vi "Lab Panel V5.40.vi"() -> ()   [LabVIEW 2017] (continued)
                          }
                        }
                      }
                    }
                  }
                }
              }
              event "RUN LAB01-2": Value Change {
                n584 = event-data() -> ("NewVal"=w850:bool)  [unwired: 1 in, 5 out]
                n585 = local write "run lab01-2"(w850) -> ()
                n586 = case shown="True" w850 {
                  tunnel: w856 -> [_ w894]
                  tunnel: w855 -> [_ w893]
                  tunnel: w853 -> [w858 w892]
                  tunnel: w854 -> [_ w891]
                  tunnel: w852 -> [_ w890]
                  tunnel: [w857 w889] -> w851
                  tunnel: w849 -> [_ w888]
                  tunnel: w848 -> [_ w887]
                  tunnel: w847 -> [_ w886]
                  tunnel: w846 -> [_ w884]
                  frame False {
                    # "stop test"
                    n587 = stacked-sequence {
                      tunnel: w858 -> [w867 _]
                      tunnel: [w859 _] -> w857
                      frame #0 {
                        n588 = local read "DISP LAB01-2"() -> (w866:T4)
                        n589 = Unbundle(w866) -> ("CYCLE"=w864:dbl, "MINS"=w865:dbl)  [unwired: 1 out]
                        n590 = case shown="\"CHART TEST\", Default" w867 {
                          tunnel: w865 -> [_ _ w874]
                          tunnel: w864 -> [w872 w873 _]
                          tunnel: [w872 w873 w874] -> w863
                          frame "CHART TEST", Default {
                          }
                          frame "CYCLE TEST" {
                          }
                          frame "T-RISE TEST" {
                          }
                        }
                        n591 = local read "TDMS LAB01-2"() -> (w871:refnum<k34>)
                        n592 = Build Array("STOPPED") -> (w868:string[])
                        n593 = Build Array(w863) -> (w862:dbl[])
                        n594 = TDMS Write(0:w871, 5:"TEST RESULT", 7:w868, 9:w862) -> (4:w860:refnum<k34>, 15:w861:errorcluster)  [unwired: 2 in, 2 out]
                        n595 = TDMS Close(8:w861, 11:w860) -> (0:w859:errorcluster)  [unwired: 1 out]
                      }
                      frame #1 {
                        n596 = local read "DISP LAB01-2"() -> (w878:T4)
                        n597 = stacked-sequence {
                          tunnel: "LAB01-2" -> [w880 w882]
                          frame #0 {
                            n598 = call "sub vi - defrag tdms v1.vi"("panel id"=w880) -> ("error out"=w879:errorcluster)  [unwired: 10 in]
                            n599 = local write "data file error"(w879) -> ()
                          }
                          frame #1 {
                            n600 = call "Save data file (stop) v3.vi"("panel id"=w882) -> ("network file save error"=w881:errorcluster)  [unwired: 9 in, 1 out]
                            n601 = local write "RESULT LAB01-2"(FALSE) -> ()
                            n602 = local write "data file error"(w881) -> ()
                          }
                        }
                        n603 = Bundle(cluster=w878, "STATUS"="STOP") -> (w876:T4)  [unwired: 2 in]
                        n604 = local write "DISP LAB01-2"(w876) -> ()
                      }
                    }
                  }
                  frame True {
                    n605 = local read "SIG LAB01-2"() -> (w885:T2)
                    n606 = stacked-sequence {
                      seq-local: [w896 _] -> [_ w900]
                      tunnel: w894 -> [_ w910]
                      tunnel: w893 -> [_ w909]
                      tunnel: w892 -> [_ w908]
                      tunnel: w891 -> [_ w907]
                      tunnel: w890 -> [_ w906]
                      tunnel: [_ w905] -> w889
                      tunnel: w888 -> [_ w904]
                      tunnel: w887 -> [_ w903]
                      tunnel: w886 -> [_ w902]
                      tunnel: w885 -> [w895 w901]
                      tunnel: w884 -> [_ w899]
                      frame #0 {
                        n607 = Unbundle(w895) -> ("AMPS"=w898:dbl)  [unwired: 4 out]
                        n608 = call "Check For Amps on v1.vi"("ID"="LAB01-2", "amps"=w898) -> ("amps"=w896:bool)  [unwired: 9 in]
                      }
                      frame #1 {
                        n609 = case shown="True" w900 {
                          tunnel: w910 -> [_ w923]
                          tunnel: w909 -> [_ w922]
                          tunnel: w908 -> [_ w921]
                          tunnel: w907 -> [_ w920]
                          tunnel: w906 -> [_ w919]
                          tunnel: [errorcluster {"status"=FALSE, "code"=0, "source"=""} ("error out") w918] -> w905
                          tunnel: w904 -> [_ w917]
                          tunnel: w903 -> [_ w916]
                          tunnel: w902 -> [_ w915]
                          tunnel: w901 -> [_ w914]
                          tunnel: w899 -> [_ w913]
                          frame False {
                            w911 = FALSE
                            n610 = local write "RUN LAB01-2"(w911) -> ()
                            n611 = local write "run lab01-2"(w911) -> ()
                          }
                          frame True {
                            n612 = stacked-sequence {
                              seq-local: [w924 _ _ _ _] -> [_ w948 _ _ _]
                              tunnel: w923 -> [w929 _ _ _ _]
                              tunnel: w922 -> [w926 _ _ _ _]
                              tunnel: w921 -> [w939 _ _ _ _]
                              tunnel: w920 -> [w932 _ _ _ _]
                              tunnel: w919 -> [w927 _ _ _ _]
                              tunnel: [_ w943 _ _ _] -> w918
                              tunnel: w917 -> [_ _ _ w970 _]
                              tunnel: w916 -> [_ _ _ w969 _]
                              tunnel: w915 -> [_ _ _ w968 _]
                              tunnel: w914 -> [_ _ _ _ _]
                              tunnel: w913 -> [_ _ _ _ w983]
                              frame #0 {
                                w925 = "\\"
                                n613 = local read "SET LAB01-2"() -> (w934:T5)
                                n614 = case shown="\"CYCLE TEST\"" w939 {
                                tunnel: ["L01-2-CHART TEST-" "L01-2-CYCLE TEST-" "L01-2-T-RISE TEST-"] -> w935
                                frame "CHART TEST", Default {
                                }
                                frame "CYCLE TEST" {
                                }
                                frame "T-RISE TEST" {
                                }
                                }
                                n615 = Unbundle(w934) -> ("DESCRIPTION"=w933:string)  [unwired: 4 out]
                                n616 = Concatenate Strings(w929, "\\", w927, w925, w926, w925) -> (w936:string)
                                n617 = String To Path(string=w936) -> (path=w938:path)
                                n618 = Concatenate Strings(w936, w935, w933, "-", w932, ".tdms") -> (w924:string)
                                n619 = Create Folder(path (use dialog)=w938) -> (error out=w937:errorcluster)  [unwired: 2 in, 2 out]
                                n620 = call <vilib>:"Clear Errors.vi"("error in (no error)"=w937) -> ()  [unwired: 5 in, 2 out]
                                n621 = global write "Global 1.vi" "LAB01-2 FILE"(w924) -> ()
                              }
                              frame #1 {
                                (unwired) FALSE
                                n622 = String To Path(string=w948) -> (path=w944:path)
                                n623 = TDMS Open(6:FALSE, 10:T22."create or replace" ("operation (0:open)"), 11:w944) -> (0:w943:errorcluster, 3:→"TDMS LAB01-2":refnum<k34>)  [unwired: 4 in]
                              }
                              frame #2 {
                                n624 = local read "SET LAB01-2"() -> (w954:T5)
                                n625 = local read "TDMS LAB01-2"() -> (w965:refnum<k34>)
                                n626 = Build Array("Testers Name", "Description", "Set Test Cycles", "T-Rise minutes", "T-Rise Deg C") -> (w955:string[])
                                n627 = Unbundle(w954) -> ("NAME"=w953:string, "DESCRIPTION"=w952:string, "CYCLES"=w951:dbl, "T-RISE mins"=w950:dbl, "T-RISE deg C"=w949:dbl)
                                n628 = Number To Decimal String(number=w951) -> (decimal integer string=w964:string)  [unwired: 1 in]
                                n629 = Number To Decimal String(number=w950) -> (decimal integer string=w963:string)  [unwired: 1 in]
                                n630 = Number To Decimal String(number=w949) -> (decimal integer string=w962:string)  [unwired: 1 in]
                                n631 = Build Array(w953, w952, w964, w963, w962) -> (w961:string[])
                                n632 = TDMS Set Properties(5:w961, 7:w955, 11:w965) -> ()  [unwired: 3 in, 4 out]
                              }
                              frame #3 {
                                n633 = local read "DISP LAB01-2"() -> (w967:T4)
                                n634 = Concatenate Strings("LAB01-2  ", w970) -> (w971:string)
                                n635 = Two Button Dialog(message=w971, 1:w968, 2:w969) -> (T button?=w973:bool)
                                n636 = case shown="True" w973 {
                                tunnel: w967 -> [w980 w981]
                                tunnel: [w980 w981] -> w977
                                tunnel: [w979 w982] -> w976
                                tunnel: [w978 w982] -> w975
                                frame False {
                                n637 = Unbundle(w980) -> ("CYCLE"=w979:dbl, "MINS"=w978:dbl)  [unwired: 1 out]
                                }
                                frame True {
                                w982 = 0.0
                                }
                                }
                                n638 = Bundle(cluster=w977, "CYCLE"=w976, "MINS"=w975, "STATUS"="RUN") -> (w966:T4)
                                n639 = local write "DISP LAB01-2"(w966) -> ()
                              }
                              frame #4 {
                                n640 = local read "TEMP START LAB01-2"() -> (w985:cluster{"TL":dbl, "TN":dbl})
                                n641 = Bundle(cluster=w985, "TL"=w983, "TN"=w983) -> (w984:cluster{"TL":dbl, "TN":dbl})
                                n642 = local write "TEMP START LAB01-2"(w984) -> ()
                              }
                            }
                          }
                        }
                      }
                    }
                  }
                }
              }
              event "RUN LAB02-1": Value Change {
                n643 = event-data() -> ("NewVal"=w991:bool)  [unwired: 1 in, 5 out]
                n644 = local read "SIG LAB02-1"() -> (w987:T2)
                n645 = case shown="True" w991 {
                  tunnel: w997 -> [_ w1035]
                  tunnel: w996 -> [_ w1034]
                  tunnel: w994 -> [w999 w1033]
                  tunnel: w995 -> [_ w1032]
                  tunnel: w993 -> [_ w1031]
                  tunnel: [w998 w1030] -> w992
                  tunnel: w990 -> [_ w1029]
                  tunnel: w989 -> [_ w1028]
                  tunnel: w988 -> [_ w1027]
                  tunnel: w987 -> [_ w1026]
                  tunnel: w986 -> [_ w1025]
                  frame False {
                    # "stop test"
                    n646 = stacked-sequence {
                      tunnel: w999 -> [w1008 _]
                      tunnel: [w1000 _] -> w998
                      frame #0 {
                        n647 = local read "DISP LAB02-1"() -> (w1007:T4)
                        n648 = Unbundle(w1007) -> ("CYCLE"=w1005:dbl, "MINS"=w1006:dbl)  [unwired: 1 out]
                        n649 = case shown="\"CYCLE TEST\"" w1008 {
                          tunnel: w1006 -> [_ _ w1015]
                          tunnel: w1005 -> [w1013 w1014 _]
                          tunnel: [w1013 w1014 w1015] -> w1004
                          frame "CHART TEST", Default {
                          }
                          frame "CYCLE TEST" {
                          }
                          frame "T-RISE TEST" {
                          }
                        }
                        n650 = local read "TDMS LAB02-1"() -> (w1012:refnum<k34>)
                        n651 = Build Array("STOPPED") -> (w1009:string[])
                        n652 = Build Array(w1004) -> (w1003:dbl[])
                        n653 = TDMS Write(0:w1012, 5:"TEST RESULT", 7:w1009, 9:w1003) -> (4:w1001:refnum<k34>, 15:w1002:errorcluster)  [unwired: 2 in, 2 out]
                        n654 = TDMS Close(8:w1002, 11:w1001) -> (0:w1000:errorcluster)  [unwired: 1 out]
                      }
                      frame #1 {
                        n655 = local read "DISP LAB02-1"() -> (w1019:T4)
                        n656 = stacked-sequence {
                          tunnel: "LAB02-1" -> [w1021 w1023]
                          frame #0 {
                            n657 = call "sub vi - defrag tdms v1.vi"("panel id"=w1021) -> ("error out"=w1020:errorcluster)  [unwired: 10 in]
                            n658 = local write "data file error"(w1020) -> ()
                          }
                          frame #1 {
                            n659 = local write "RESULT LAB02-1"(FALSE) -> ()
                            n660 = call "Save data file (stop) v3.vi"("panel id"=w1023) -> ("network file save error"=w1022:errorcluster)  [unwired: 9 in, 1 out]
                            n661 = local write "data file error"(w1022) -> ()
                          }
                        }
                        n662 = Bundle(cluster=w1019, "STATUS"="STOP") -> (w1017:T4)  [unwired: 2 in]
                        n663 = local write "DISP LAB02-1"(w1017) -> ()
                      }
                    }
                  }
                  frame True {
                    n664 = stacked-sequence {
                      seq-local: [w1037 _] -> [_ w1041]
                      tunnel: w1035 -> [_ w1051]
                      tunnel: w1034 -> [_ w1050]
                      tunnel: w1033 -> [_ w1049]
                      tunnel: w1032 -> [_ w1048]
                      tunnel: w1031 -> [_ w1047]
                      tunnel: [_ w1046] -> w1030
                      tunnel: w1029 -> [_ w1045]
                      tunnel: w1028 -> [_ w1044]
                      tunnel: w1027 -> [_ w1043]
                      tunnel: w1026 -> [w1036 w1042]
                      tunnel: w1025 -> [_ w1040]
                      frame #0 {
                        n665 = Unbundle(w1036) -> ("AMPS"=w1039:dbl)  [unwired: 4 out]
                        n666 = call "Check For Amps on v1.vi"("ID"="LAB02-1", "amps"=w1039) -> ("amps"=w1037:bool)  [unwired: 9 in]
                      }
                      frame #1 {
                        n667 = case shown="True" w1041 {
                          tunnel: w1051 -> [_ w1064]
                          tunnel: w1050 -> [_ w1063]
                          tunnel: w1049 -> [_ w1062]
                          tunnel: w1048 -> [_ w1061]
                          tunnel: w1047 -> [_ w1060]
                          tunnel: [errorcluster {"status"=FALSE, "code"=0, "source"=""} ("error out") w1059] -> w1046
                          tunnel: w1045 -> [_ w1058]
                          tunnel: w1044 -> [_ w1057]
                          tunnel: w1043 -> [_ w1056]
                          tunnel: w1042 -> [_ w1055]
                          tunnel: w1040 -> [_ w1054]
                          frame False {
                            w1053 = FALSE
                            n668 = local write "RUN LAB02-1"(w1053) -> ()
                            n669 = local write "run lab02-1"(w1053) -> ()
                          }
                          frame True {
                            n670 = stacked-sequence {
                              seq-local: [w1065 _ _ _ _] -> [_ w1089 _ _ _]
                              tunnel: w1064 -> [w1070 _ _ _ _]
                              tunnel: w1063 -> [w1067 _ _ _ _]
                              tunnel: w1062 -> [w1080 _ _ _ _]
                              tunnel: w1061 -> [w1073 _ _ _ _]
                              tunnel: w1060 -> [w1068 _ _ _ _]
                              tunnel: [_ w1084 _ _ _] -> w1059
                              tunnel: w1058 -> [_ _ _ w1110 _]
                              tunnel: w1057 -> [_ _ _ w1109 _]
                              tunnel: w1056 -> [_ _ _ w1108 _]
                              tunnel: w1055 -> [_ _ _ _ _]
                              tunnel: w1054 -> [_ _ _ _ w1124]
                              frame #0 {
                                w1066 = "\\"
                                n671 = local read "SET LAB02-1"() -> (w1075:T5)
                                n672 = case shown="\"CYCLE TEST\"" w1080 {
                                tunnel: ["L02-1-CHART TEST-" "L02-1-CYCLE TEST-" "L02-1-T-RISE TEST-"] -> w1076
                                frame "CHART TEST", Default {
                                }
                                frame "CYCLE TEST" {
                                }
                                frame "T-RISE TEST" {
                                }
                                }
                                n673 = Unbundle(w1075) -> ("DESCRIPTION"=w1074:string)  [unwired: 4 out]
                                n674 = Concatenate Strings(w1070, "\\", w1068, w1066, w1067, w1066) -> (w1077:string)
                                n675 = String To Path(string=w1077) -> (path=w1079:path)
                                n676 = Concatenate Strings(w1077, w1076, w1074, "-", w1073, ".tdms") -> (w1065:string)
                                n677 = Create Folder(path (use dialog)=w1079) -> (error out=w1078:errorcluster)  [unwired: 2 in, 2 out]
                                n678 = global write "Global 1.vi" "LAB02-1 FILE"(w1065) -> ()
                                n679 = call <vilib>:"Clear Errors.vi"("error in (no error)"=w1078) -> ()  [unwired: 5 in, 2 out]
                              }
                              frame #1 {
                                (unwired) FALSE
                                n680 = String To Path(string=w1089) -> (path=w1085:path)
                                n681 = TDMS Open(6:FALSE, 10:T22."create or replace" ("operation (0:open)"), 11:w1085) -> (0:w1084:errorcluster, 3:→"TDMS LAB02-1":refnum<k34>)  [unwired: 4 in]
                              }
                              frame #2 {
                                n682 = local read "SET LAB02-1"() -> (w1095:T5)
                                n683 = local read "TDMS LAB02-1"() -> (w1106:refnum<k34>)
                                n684 = Build Array("Testers Name", "Description", "Set Test Cycles", "T-Rise minutes", "T-Rise Deg C") -> (w1096:string[])
                                n685 = Unbundle(w1095) -> ("NAME"=w1094:string, "DESCRIPTION"=w1093:string, "CYCLES"=w1092:dbl, "T-RISE mins"=w1091:dbl, "T-RISE deg C"=w1090:dbl)
                                n686 = Number To Decimal String(number=w1092) -> (decimal integer string=w1105:string)  [unwired: 1 in]
                                n687 = Number To Decimal String(number=w1091) -> (decimal integer string=w1104:string)  [unwired: 1 in]
                                n688 = Number To Decimal String(number=w1090) -> (decimal integer string=w1103:string)  [unwired: 1 in]
                                n689 = Build Array(w1094, w1093, w1105, w1104, w1103) -> (w1102:string[])
                                n690 = TDMS Set Properties(5:w1102, 7:w1096, 11:w1106) -> ()  [unwired: 3 in, 4 out]
                              }
                              frame #3 {
                                n691 = local read "DISP LAB02-1"() -> (w1111:T4)
                                n692 = Concatenate Strings("LAB02-1  ", w1110) -> (w1112:string)
                                n693 = Two Button Dialog(message=w1112, 1:w1108, 2:w1109) -> (T button?=w1114:bool)
                                n694 = case shown="True" w1114 {
                                tunnel: w1111 -> [w1121 w1122]
                                tunnel: [w1121 w1122] -> w1118
                                tunnel: [w1120 w1123] -> w1117
                                tunnel: [w1119 w1123] -> w1116
                                frame False {
                                n695 = Unbundle(w1121) -> ("CYCLE"=w1120:dbl, "MINS"=w1119:dbl)  [unwired: 1 out]
                                }
                                frame True {
                                w1123 = 0.0
                                }
                                }
                                n696 = Bundle(cluster=w1118, "CYCLE"=w1117, "MINS"=w1116, "STATUS"="RUN") -> (w1107:T4)
                                n697 = local write "DISP LAB02-1"(w1107) -> ()
                              }
                              frame #4 {
                                n698 = local read "TEMP START LAB02-1"() -> (w1126:cluster{"TL":dbl, "TN":dbl})
                                n699 = Bundle(cluster=w1126, "TL"=w1124, "TN"=w1124) -> (w1125:cluster{"TL":dbl, "TN":dbl})
                                n700 = local write "TEMP START LAB02-1"(w1125) -> ()
                              }
                            }
                          }
                        }
                      }
                    }
                  }
                }
                n701 = local write "run lab02-1"(w991) -> ()
              }
              event "RUN LAB02-2": Value Change {
                n702 = event-data() -> ("NewVal"=w1131:bool)  [unwired: 1 in, 5 out]
                n703 = local write "run lab02-2"(w1131) -> ()
                n704 = case shown="True" w1131 {
                  tunnel: w1137 -> [_ w1175]
                  tunnel: w1136 -> [_ w1174]
                  tunnel: w1134 -> [w1139 w1173]
                  tunnel: w1135 -> [_ w1172]
                  tunnel: w1133 -> [_ w1171]
                  tunnel: [w1138 w1170] -> w1132
                  tunnel: w1130 -> [_ w1169]
                  tunnel: w1129 -> [_ w1168]
                  tunnel: w1128 -> [_ w1167]
                  tunnel: w1127 -> [_ w1165]
                  frame False {
                    # "stop test"
                    n705 = stacked-sequence {
                      tunnel: w1139 -> [w1148 _]
                      tunnel: [w1140 _] -> w1138
                      frame #0 {
                        n706 = local read "DISP LAB02-2"() -> (w1147:T4)
                        n707 = Unbundle(w1147) -> ("CYCLE"=w1145:dbl, "MINS"=w1146:dbl)  [unwired: 1 out]
                        n708 = case shown="\"CYCLE TEST\"" w1148 {
                          tunnel: w1146 -> [_ _ w1155]
                          tunnel: w1145 -> [w1153 w1154 _]
                          tunnel: [w1153 w1154 w1155] -> w1144
                          frame "CHART TEST", Default {
                          }
                          frame "CYCLE TEST" {
                          }
                          frame "T-RISE TEST" {
                          }
                        }
                        n709 = local read "TDMS LAB02-2"() -> (w1152:refnum<k34>)
                        n710 = Build Array("STOPPED") -> (w1149:string[])
                        n711 = Build Array(w1144) -> (w1143:dbl[])
                        n712 = TDMS Write(0:w1152, 5:"TEST RESULT", 7:w1149, 9:w1143) -> (4:w1141:refnum<k34>, 15:w1142:errorcluster)  [unwired: 2 in, 2 out]
                        n713 = TDMS Close(8:w1142, 11:w1141) -> (0:w1140:errorcluster)  [unwired: 1 out]
                      }
                      frame #1 {
                        n714 = local read "DISP LAB02-2"() -> (w1159:T4)
                        n715 = stacked-sequence {
                          tunnel: "LAB02-2" -> [w1161 w1163]
                          frame #0 {
                            n716 = call "sub vi - defrag tdms v1.vi"("panel id"=w1161) -> ("error out"=w1160:errorcluster)  [unwired: 10 in]
                            n717 = local write "data file error"(w1160) -> ()
                          }
                          frame #1 {
                            n718 = call "Save data file (stop) v3.vi"("panel id"=w1163) -> ("network file save error"=w1162:errorcluster)  [unwired: 9 in, 1 out]
                            n719 = local write "RESULT LAB02-2"(FALSE) -> ()
                            n720 = local write "data file error"(w1162) -> ()
                          }
                        }
                        n721 = Bundle(cluster=w1159, "STATUS"="STOP") -> (w1157:T4)  [unwired: 2 in]
                        n722 = local write "DISP LAB02-2"(w1157) -> ()
                      }
                    }
                  }
                  frame True {
                    n723 = local read "SIG LAB02-2"() -> (w1166:T2)
                    n724 = stacked-sequence {
                      seq-local: [w1177 _] -> [_ w1181]
                      tunnel: w1175 -> [_ w1191]
                      tunnel: w1174 -> [_ w1190]
                      tunnel: w1173 -> [_ w1189]
                      tunnel: w1172 -> [_ w1188]
                      tunnel: w1171 -> [_ w1187]
                      tunnel: [_ w1186] -> w1170
                      tunnel: w1169 -> [_ w1185]
                      tunnel: w1168 -> [_ w1184]
                      tunnel: w1167 -> [_ w1183]
                      tunnel: w1166 -> [w1176 w1182]
                      tunnel: w1165 -> [_ w1180]
                      frame #0 {
                        n725 = Unbundle(w1176) -> ("AMPS"=w1179:dbl)  [unwired: 4 out]
                        n726 = call "Check For Amps on v1.vi"("ID"="LAB02-2", "amps"=w1179) -> ("amps"=w1177:bool)  [unwired: 9 in]
                      }
                      frame #1 {
                        n727 = case shown="True" w1181 {
                          tunnel: w1191 -> [_ w1204]
                          tunnel: w1190 -> [_ w1203]
                          tunnel: w1189 -> [_ w1202]
                          tunnel: w1188 -> [_ w1201]
                          tunnel: w1187 -> [_ w1200]
                          tunnel: [errorcluster {"status"=FALSE, "code"=0, "source"=""} ("error out") w1199] -> w1186
                          tunnel: w1185 -> [_ w1198]
                          tunnel: w1184 -> [_ w1197]
                          tunnel: w1183 -> [_ w1196]
                          tunnel: w1182 -> [_ w1195]
                          tunnel: w1180 -> [_ w1194]
                          frame False {
                            w1192 = FALSE
                            n728 = local write "RUN LAB02-2"(w1192) -> ()
                            n729 = local write "run lab02-2"(w1192) -> ()
                          }
                          frame True {
                            n730 = stacked-sequence {
                              seq-local: [w1205 _ _ _ _] -> [_ w1229 _ _ _]
                              tunnel: w1204 -> [w1210 _ _ _ _]
                              tunnel: w1203 -> [w1207 _ _ _ _]
                              tunnel: w1202 -> [w1220 _ _ _ _]
                              tunnel: w1201 -> [w1213 _ _ _ _]
                              tunnel: w1200 -> [w1208 _ _ _ _]
                              tunnel: [_ w1224 _ _ _] -> w1199
                              tunnel: w1198 -> [_ _ _ w1250 _]
                              tunnel: w1197 -> [_ _ _ w1249 _]
                              tunnel: w1196 -> [_ _ _ w1248 _]
                              tunnel: w1195 -> [_ _ _ _ _]
                              tunnel: w1194 -> [_ _ _ _ w1264]
                              frame #0 {
                                w1206 = "\\"
                                n731 = local read "SET LAB02-2"() -> (w1215:T5)
                                n732 = case shown="\"CYCLE TEST\"" w1220 {
                                tunnel: ["L02-2-CHART TEST-" "L02-2-CYCLE TEST-" "L02-2-T-RISE TEST-"] -> w1216
                                frame "CHART TEST", Default {
                                }
                                frame "CYCLE TEST" {
                                }
                                frame "T-RISE TEST" {
                                }
                                }
                                n733 = Unbundle(w1215) -> ("DESCRIPTION"=w1214:string)  [unwired: 4 out]
                                n734 = Concatenate Strings(w1210, "\\", w1208, w1206, w1207, w1206) -> (w1217:string)
                                n735 = String To Path(string=w1217) -> (path=w1219:path)
                                n736 = Concatenate Strings(w1217, w1216, w1214, "-", w1213, ".tdms") -> (w1205:string)
                                n737 = Create Folder(path (use dialog)=w1219) -> (error out=w1218:errorcluster)  [unwired: 2 in, 2 out]
                                n738 = global write "Global 1.vi" "LAB02-2 FILE"(w1205) -> ()
                                n739 = call <vilib>:"Clear Errors.vi"("error in (no error)"=w1218) -> ()  [unwired: 5 in, 2 out]
                              }
                              frame #1 {
                                (unwired) FALSE
                                n740 = String To Path(string=w1229) -> (path=w1225:path)
                                n741 = TDMS Open(6:FALSE, 10:T22."create or replace" ("operation (0:open)"), 11:w1225) -> (0:w1224:errorcluster, 3:→"TDMS LAB02-2":refnum<k34>)  [unwired: 4 in]
                              }
                              frame #2 {
                                n742 = local read "SET LAB02-2"() -> (w1235:T5)
                                n743 = local read "TDMS LAB02-2"() -> (w1246:refnum<k34>)
                                n744 = Build Array("Testers Name", "Description", "Set Test Cycles", "T-Rise minutes", "T-Rise Deg C") -> (w1236:string[])
                                n745 = Unbundle(w1235) -> ("NAME"=w1234:string, "DESCRIPTION"=w1233:string, "CYCLES"=w1232:dbl, "T-RISE mins"=w1231:dbl, "T-RISE deg C"=w1230:dbl)
                                n746 = Number To Decimal String(number=w1232) -> (decimal integer string=w1245:string)  [unwired: 1 in]
                                n747 = Number To Decimal String(number=w1231) -> (decimal integer string=w1244:string)  [unwired: 1 in]
                                n748 = Number To Decimal String(number=w1230) -> (decimal integer string=w1243:string)  [unwired: 1 in]
                                n749 = Build Array(w1234, w1233, w1245, w1244, w1243) -> (w1242:string[])
                                n750 = TDMS Set Properties(5:w1242, 7:w1236, 11:w1246) -> ()  [unwired: 3 in, 4 out]
                              }
                              frame #3 {
                                n751 = local read "DISP LAB02-2"() -> (w1251:T4)
                                n752 = Concatenate Strings("LAB02-2  ", w1250) -> (w1252:string)
                                n753 = Two Button Dialog(message=w1252, 1:w1248, 2:w1249) -> (T button?=w1254:bool)
                                n754 = case shown="True" w1254 {
                                tunnel: w1251 -> [w1261 w1262]
                                tunnel: [w1261 w1262] -> w1258
                                tunnel: [w1260 w1263] -> w1257
                                tunnel: [w1259 w1263] -> w1256
                                frame False {
                                n755 = Unbundle(w1261) -> ("CYCLE"=w1260:dbl, "MINS"=w1259:dbl)  [unwired: 1 out]
                                }
                                frame True {
                                w1263 = 0.0
                                }
                                }
                                n756 = Bundle(cluster=w1258, "CYCLE"=w1257, "MINS"=w1256, "STATUS"="RUN") -> (w1247:T4)
                                n757 = local write "DISP LAB02-2"(w1247) -> ()
                              }
                              frame #4 {
                                n758 = local read "TEMP START LAB02-2"() -> (w1266:cluster{"TL":dbl, "TN":dbl})
                                n759 = Bundle(cluster=w1266, "TL"=w1264, "TN"=w1264) -> (w1265:cluster{"TL":dbl, "TN":dbl})
                                n760 = local write "TEMP START LAB02-2"(w1265) -> ()
                              }
                            }
                          }
                        }
                      }
                    }
                  }
                }
              }
              event "RUN LAB03-1": Value Change {
                n761 = event-data() -> ("NewVal"=w1271:bool)  [unwired: 1 in, 5 out]
                n762 = local write "run lab03-1"(w1271) -> ()
                n763 = case shown="True" w1271 {
                  tunnel: w1277 -> [_ w1315]
                  tunnel: w1276 -> [_ w1314]
                  tunnel: w1274 -> [w1279 w1313]
                  tunnel: w1275 -> [_ w1312]
                  tunnel: w1273 -> [_ w1311]
                  tunnel: [w1278 w1310] -> w1272
                  tunnel: w1270 -> [_ w1309]
                  tunnel: w1269 -> [_ w1308]
                  tunnel: w1268 -> [_ w1307]
                  tunnel: w1267 -> [_ w1305]
                  frame False {
                    # "stop test"
                    n764 = stacked-sequence {
                      tunnel: w1279 -> [w1288 _]
                      tunnel: [w1280 _] -> w1278
                      frame #0 {
                        n765 = local read "DISP LAB03-1"() -> (w1287:T4)
                        n766 = Unbundle(w1287) -> ("CYCLE"=w1285:dbl, "MINS"=w1286:dbl)  [unwired: 1 out]
                        n767 = case shown="\"CYCLE TEST\"" w1288 {
                          tunnel: w1286 -> [_ _ w1295]
                          tunnel: w1285 -> [w1293 w1294 _]
                          tunnel: [w1293 w1294 w1295] -> w1284
                          frame "CHART TEST", Default {
                          }
                          frame "CYCLE TEST" {
                          }
                          frame "T-RISE TEST" {
                          }
                        }
                        n768 = local read "TDMS LAB03-1"() -> (w1292:refnum<k34>)
                        n769 = Build Array("STOPPED") -> (w1289:string[])
                        n770 = Build Array(w1284) -> (w1283:dbl[])
                        n771 = TDMS Write(0:w1292, 5:"TEST RESULT", 7:w1289, 9:w1283) -> (4:w1281:refnum<k34>, 15:w1282:errorcluster)  [unwired: 2 in, 2 out]
                        n772 = TDMS Close(8:w1282, 11:w1281) -> (0:w1280:errorcluster)  [unwired: 1 out]
                      }
                      frame #1 {
                        n773 = local read "DISP LAB03-1"() -> (w1299:T4)
                        n774 = stacked-sequence {
                          tunnel: "LAB03-1" -> [w1301 w1303]
                          frame #0 {
                            n775 = call "sub vi - defrag tdms v1.vi"("panel id"=w1301) -> ("error out"=w1300:errorcluster)  [unwired: 10 in]
                            n776 = local write "data file error"(w1300) -> ()
                          }
                          frame #1 {
                            n777 = call "Save data file (stop) v3.vi"("panel id"=w1303) -> ("network file save error"=w1302:errorcluster)  [unwired: 9 in, 1 out]
                            n778 = local write "RESULT LAB03-1"(FALSE) -> ()
                            n779 = local write "data file error"(w1302) -> ()
                          }
                        }
                        n780 = Bundle(cluster=w1299, "STATUS"="STOP") -> (w1297:T4)  [unwired: 2 in]
                        n781 = local write "DISP LAB03-1"(w1297) -> ()
                      }
                    }
                  }
                  frame True {
                    n782 = local read "SIG LAB03-1"() -> (w1306:T2)
                    n783 = stacked-sequence {
                      seq-local: [w1317 _] -> [_ w1321]
                      tunnel: w1315 -> [_ w1331]
                      tunnel: w1314 -> [_ w1330]
                      tunnel: w1313 -> [_ w1329]
                      tunnel: w1312 -> [_ w1328]
                      tunnel: w1311 -> [_ w1327]
                      tunnel: [_ w1326] -> w1310
                      tunnel: w1309 -> [_ w1325]
                      tunnel: w1308 -> [_ w1324]
                      tunnel: w1307 -> [_ w1323]
                      tunnel: w1306 -> [w1316 w1322]
                      tunnel: w1305 -> [_ w1320]
                      frame #0 {
                        n784 = Unbundle(w1316) -> ("AMPS"=w1319:dbl)  [unwired: 4 out]
                        n785 = call "Check For Amps on v1.vi"("ID"="LAB03-1", "amps"=w1319) -> ("amps"=w1317:bool)  [unwired: 9 in]
                      }
                      frame #1 {
                        n786 = case shown="True" w1321 {
                          tunnel: w1331 -> [_ w1344]
                          tunnel: w1330 -> [_ w1343]
                          tunnel: w1329 -> [_ w1342]
                          tunnel: w1328 -> [_ w1341]
                          tunnel: w1327 -> [_ w1340]
                          tunnel: [errorcluster {"status"=FALSE, "code"=0, "source"=""} ("error out") w1339] -> w1326
                          tunnel: w1325 -> [_ w1338]
                          tunnel: w1324 -> [_ w1337]
                          tunnel: w1323 -> [_ w1336]
                          tunnel: w1322 -> [_ w1335]
                          tunnel: w1320 -> [_ w1334]
                          frame False {
                            w1332 = FALSE
                            n787 = local write "RUN LAB03-1"(w1332) -> ()
                            n788 = local write "run lab03-1"(w1332) -> ()
                          }
                          frame True {
                            n789 = stacked-sequence {
                              seq-local: [w1345 _ _ _ _] -> [_ w1369 _ _ _]
                              tunnel: w1344 -> [w1350 _ _ _ _]
                              tunnel: w1343 -> [w1347 _ _ _ _]
                              tunnel: w1342 -> [w1360 _ _ _ _]
                              tunnel: w1341 -> [w1353 _ _ _ _]
                              tunnel: w1340 -> [w1348 _ _ _ _]
                              tunnel: [_ w1364 _ _ _] -> w1339
                              tunnel: w1338 -> [_ _ _ w1389 _]
                              tunnel: w1337 -> [_ _ _ w1388 _]
                              tunnel: w1336 -> [_ _ _ w1387 _]
                              tunnel: w1335 -> [_ _ _ _ _]
                              tunnel: w1334 -> [_ _ _ _ w1404]
                              frame #0 {
                                w1346 = "\\"
                                n790 = local read "SET LAB03-1"() -> (w1355:T5)
                                n791 = case shown="\"T-RISE TEST\"" w1360 {
                                tunnel: ["L03-1-CHART TEST-" "L03-1-CYCLE TEST-" "L03-1-T-RISE TEST-"] -> w1356
                                frame "CHART TEST", Default {
                                }
                                frame "CYCLE TEST" {
                                }
                                frame "T-RISE TEST" {
                                }
                                }
                                n792 = Unbundle(w1355) -> ("DESCRIPTION"=w1354:string)  [unwired: 4 out]
                                n793 = Concatenate Strings(w1350, "\\", w1348, w1346, w1347, w1346) -> (w1357:string)
                                n794 = String To Path(string=w1357) -> (path=w1359:path)
                                n795 = Concatenate Strings(w1357, w1356, w1354, "-", w1353, ".tdms") -> (w1345:string)
                                n796 = Create Folder(path (use dialog)=w1359) -> (error out=w1358:errorcluster)  [unwired: 2 in, 2 out]
                                n797 = global write "Global 1.vi" "LAB03-1 FILE"(w1345) -> ()
                                n798 = call <vilib>:"Clear Errors.vi"("error in (no error)"=w1358) -> ()  [unwired: 5 in, 2 out]
                              }
                              frame #1 {
                                (unwired) FALSE
                                n799 = String To Path(string=w1369) -> (path=w1365:path)
                                n800 = TDMS Open(6:FALSE, 10:T22."create or replace" ("operation (0:open)"), 11:w1365) -> (0:w1364:errorcluster, 3:→"TDMS LAB03-1":refnum<k34>)  [unwired: 4 in]
                              }
                              frame #2 {
                                n801 = local read "SET LAB03-1"() -> (w1375:T5)
                                n802 = local read "TDMS LAB03-1"() -> (w1386:refnum<k34>)
                                n803 = Build Array("Testers Name", "Description", "Set Test Cycles", "T-Rise minutes", "T-Rise Deg C") -> (w1376:string[])
                                n804 = Unbundle(w1375) -> ("NAME"=w1374:string, "DESCRIPTION"=w1373:string, "CYCLES"=w1372:dbl, "T-RISE mins"=w1371:dbl, "T-RISE deg C"=w1370:dbl)
                                n805 = Number To Decimal String(number=w1372) -> (decimal integer string=w1385:string)  [unwired: 1 in]
                                n806 = Number To Decimal String(number=w1371) -> (decimal integer string=w1384:string)  [unwired: 1 in]
                                n807 = Number To Decimal String(number=w1370) -> (decimal integer string=w1383:string)  [unwired: 1 in]
                                n808 = Build Array(w1374, w1373, w1385, w1384, w1383) -> (w1382:string[])
                                n809 = TDMS Set Properties(5:w1382, 7:w1376, 11:w1386) -> ()  [unwired: 3 in, 4 out]
                              }
                              frame #3 {
                                n810 = local read "DISP LAB03-1"() -> (w1391:T4)
                                n811 = Concatenate Strings("LAB03-1  ", w1389) -> (w1392:string)
                                n812 = Two Button Dialog(message=w1392, 1:w1387, 2:w1388) -> (T button?=w1394:bool)
                                n813 = case shown="True" w1394 {
                                tunnel: w1391 -> [w1401 w1402]
                                tunnel: [w1401 w1402] -> w1398
                                tunnel: [w1400 w1403] -> w1397
                                tunnel: [w1399 w1403] -> w1396
                                frame False {
                                n814 = Unbundle(w1401) -> ("CYCLE"=w1400:dbl, "MINS"=w1399:dbl)  [unwired: 1 out]
                                }
                                frame True {
                                w1403 = 0.0
                                }
                                }
                                n815 = Bundle(cluster=w1398, "CYCLE"=w1397, "MINS"=w1396, "STATUS"="RUN") -> (w1390:T4)
                                n816 = local write "DISP LAB03-1"(w1390) -> ()
                              }
                              frame #4 {
                                n817 = local read "TEMP START LAB03-1"() -> (w1406:cluster{"TL":dbl, "TN":dbl})
                                n818 = Bundle(cluster=w1406, "TL"=w1404, "TN"=w1404) -> (w1405:cluster{"TL":dbl, "TN":dbl})
                                n819 = local write "TEMP START LAB03-1"(w1405) -> ()
                              }
                            }
                          }
                        }
                      }
                    }
                  }
                }
              }
              event "RUN LAB03-2": Value Change {
                n820 = event-data() -> ("NewVal"=w1411:bool)  [unwired: 1 in, 5 out]
                n821 = local write "run lab03-2"(w1411) -> ()
                n822 = case shown="True" w1411 {
                  tunnel: w1417 -> [_ w1455]
                  tunnel: w1416 -> [_ w1454]
                  tunnel: w1414 -> [w1419 w1453]
                  tunnel: w1415 -> [_ w1452]
                  tunnel: w1413 -> [_ w1451]
                  tunnel: [w1418 w1450] -> w1412
                  tunnel: w1410 -> [_ w1449]
                  tunnel: w1409 -> [_ w1448]
                  tunnel: w1408 -> [_ w1447]
                  tunnel: w1407 -> [_ w1445]
                  frame False {
                    # "stop test"
                    n823 = stacked-sequence {
                      tunnel: w1419 -> [w1428 _]
                      tunnel: [w1420 _] -> w1418
                      frame #0 {
                        n824 = local read "DISP LAB03-2"() -> (w1427:T4)
                        n825 = Unbundle(w1427) -> ("CYCLE"=w1425:dbl, "MINS"=w1426:dbl)  [unwired: 1 out]
                        n826 = case shown="\"CYCLE TEST\"" w1428 {
                          tunnel: w1426 -> [_ _ w1435]
                          tunnel: w1425 -> [w1433 w1434 _]
                          tunnel: [w1433 w1434 w1435] -> w1424
                          frame "CHART TEST", Default {
                          }
                          frame "CYCLE TEST" {
                          }
                          frame "T-RISE TEST" {
                          }
                        }
                        n827 = local read "TDMS LAB03-2"() -> (w1432:refnum<k34>)
                        n828 = Build Array("STOPPED") -> (w1429:string[])
                        n829 = Build Array(w1424) -> (w1423:dbl[])
                        n830 = TDMS Write(0:w1432, 5:"TEST RESULT", 7:w1429, 9:w1423) -> (4:w1421:refnum<k34>, 15:w1422:errorcluster)  [unwired: 2 in, 2 out]
                        n831 = TDMS Close(8:w1422, 11:w1421) -> (0:w1420:errorcluster)  [unwired: 1 out]
                      }
                      frame #1 {
                        n832 = local read "DISP LAB03-2"() -> (w1439:T4)
                        n833 = stacked-sequence {
                          tunnel: "LAB03-2" -> [w1441 w1443]
                          frame #0 {
                            n834 = call "sub vi - defrag tdms v1.vi"("panel id"=w1441) -> ("error out"=w1440:errorcluster)  [unwired: 10 in]
                            n835 = local write "data file error"(w1440) -> ()
                          }
                          frame #1 {
                            n836 = call "Save data file (stop) v3.vi"("panel id"=w1443) -> ("network file save error"=w1442:errorcluster)  [unwired: 9 in, 1 out]
                            n837 = local write "RESULT LAB03-2"(FALSE) -> ()
                            n838 = local write "data file error"(w1442) -> ()
                          }
                        }
                        n839 = Bundle(cluster=w1439, "STATUS"="STOP") -> (w1437:T4)  [unwired: 2 in]
                        n840 = local write "DISP LAB03-2"(w1437) -> ()
                      }
                    }
                  }
                  frame True {
                    n841 = local read "SIG LAB03-2"() -> (w1446:T2)
                    n842 = stacked-sequence {
                      seq-local: [w1457 _] -> [_ w1461]
                      tunnel: w1455 -> [_ w1471]
                      tunnel: w1454 -> [_ w1470]
                      tunnel: w1453 -> [_ w1469]
                      tunnel: w1452 -> [_ w1468]
                      tunnel: w1451 -> [_ w1467]
                      tunnel: [_ w1466] -> w1450
                      tunnel: w1449 -> [_ w1465]
                      tunnel: w1448 -> [_ w1464]
                      tunnel: w1447 -> [_ w1463]
                      tunnel: w1446 -> [w1456 w1462]
                      tunnel: w1445 -> [_ w1460]
                      frame #0 {
                        n843 = Unbundle(w1456) -> ("AMPS"=w1459:dbl)  [unwired: 4 out]
                        n844 = call "Check For Amps on v1.vi"("ID"="LAB03-2", "amps"=w1459) -> ("amps"=w1457:bool)  [unwired: 9 in]
                      }
                      frame #1 {
                        n845 = case shown="True" w1461 {
                          tunnel: w1471 -> [_ w1484]
                          tunnel: w1470 -> [_ w1483]
                          tunnel: w1469 -> [_ w1482]
                          tunnel: w1468 -> [_ w1481]
                          tunnel: w1467 -> [_ w1480]
                          tunnel: [errorcluster {"status"=FALSE, "code"=0, "source"=""} ("error out") w1479] -> w1466
                          tunnel: w1465 -> [_ w1478]
                          tunnel: w1464 -> [_ w1477]
                          tunnel: w1463 -> [_ w1476]
                          tunnel: w1462 -> [_ w1475]
                          tunnel: w1460 -> [_ w1474]
                          frame False {
                            w1472 = FALSE
                            n846 = local write "RUN LAB03-2"(w1472) -> ()
                            n847 = local write "run lab03-2"(w1472) -> ()
                          }
                          frame True {
                            n848 = stacked-sequence {
                              seq-local: [w1485 _ _ _ _] -> [_ w1509 _ _ _]
                              tunnel: w1484 -> [w1490 _ _ _ _]
                              tunnel: w1483 -> [w1487 _ _ _ _]
                              tunnel: w1482 -> [w1500 _ _ _ _]
                              tunnel: w1481 -> [w1493 _ _ _ _]
                              tunnel: w1480 -> [w1488 _ _ _ _]
                              tunnel: [_ w1504 _ _ _] -> w1479
                              tunnel: w1478 -> [_ _ _ w1530 _]
                              tunnel: w1477 -> [_ _ _ w1529 _]
                              tunnel: w1476 -> [_ _ _ w1528 _]
                              tunnel: w1475 -> [_ _ _ _ _]
                              tunnel: w1474 -> [_ _ _ _ w1544]
                              frame #0 {
                                w1486 = "\\"
                                n849 = local read "SET LAB03-2"() -> (w1495:T5)
                                n850 = case shown="\"T-RISE TEST\"" w1500 {
                                tunnel: ["L03-2-CHART TEST-" "L03-2-CYCLE TEST-" "L03-2-T-RISE TEST-"] -> w1496
